vi "jsontest3.vi"() -> ()   [LabVIEW 2014]
panel:
  out "JSON string":string
  out "value 3":T1(array[cluster])
  in  "value 2":T1(array[cluster])=[{"DEPT"="Z", "LINE"="L2A", "STANO"="1", "WORKNO"="壓縮機", "PRODSN"="0DO1100587", "COMPNTID"="9SS064XGA21", "COMPNTLOT"="F0033", "COMPNTSN"="9SS064XGA21~20210520F0033949", "USEDQTY"=1, "OPDATE"="20211026082804", "OPUSER"="SYSTEM", "RECVDATE"="20211026082804", "MMODU"="KCI"}, {"DEPT"="Z", "LINE"="L2A", "STANO"="1", "WORKNO"="馬達", "PRODSN"="0DO1100587", "COMPNTID"="9SS064XGA21", "COMPNTLOT"="F0033", "COMPNTSN"="9SS064XGA21", "USEDQTY"=1, "OPDATE"="202110260828", "OPUSER"="SYSTEM", "RECVDATE"="202110260828", "MMODU"="KCI"}, {"DEPT"="Z", "LINE"="L2A", "STANO"="1", "WORKNO"="電源板", "PRODSN"="0DO1100587", "COMPNTID"="2", "COMPNTLOT"="3", "COMPNTSN"="4", "USEDQTY"=1, "OPDATE"="202110260828", "OPUSER"="SYSTEM", "RECVDATE"="202110260828", "MMODU"="KCI"}]
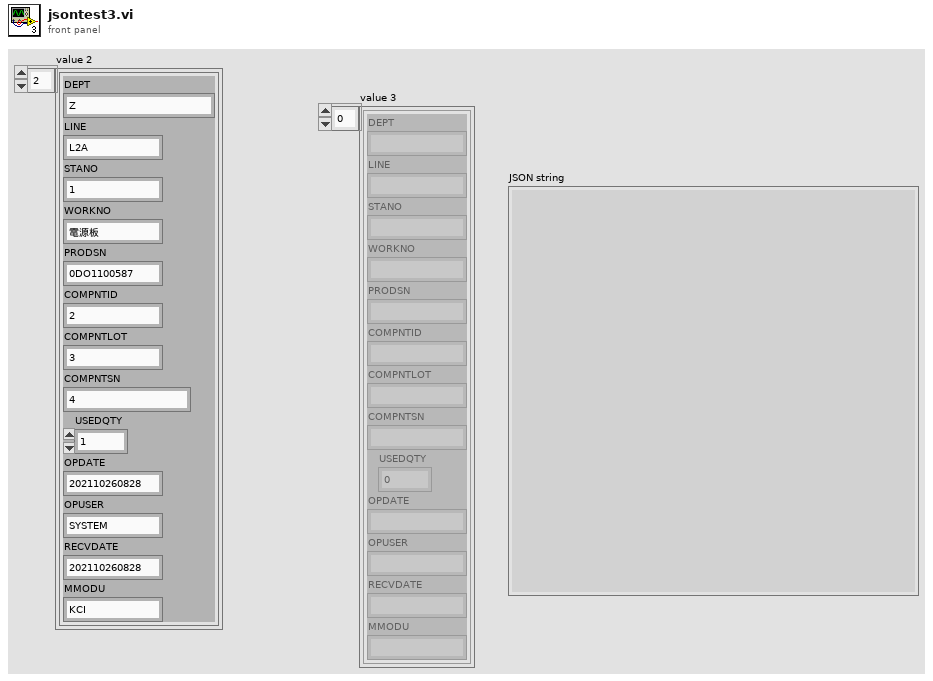
[diagram p1: front panel]
types:
  T1 = cluster{"DEPT":string, "LINE":string, "STANO":string, "WORKNO":string, "PRODSN":string, "COMPNTID":string, "COMPNTLOT":string, "COMPNTSN":string, "USEDQTY":i16, "OPDATE":string, "OPUSER":string, "RECVDATE":string, "MMODU":string}[]
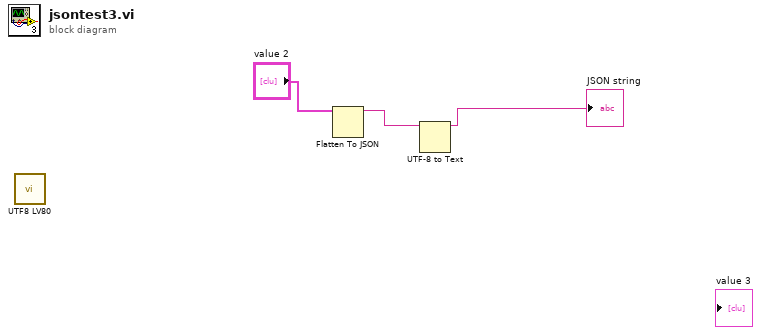
[diagram p0: block diagram]
diagram:
  n1 = call "UTF8 LV80.vi"() -> ()  [unwired: 1 in]
  n2 = Flatten To JSON(anything="value 2") -> (JSON string=w2:string)  [unwired: 2 in, 1 out]
  n3 = UTF-8 to Text(11:w2) -> (3:→"JSON string":string)  [unwired: 2 in, 1 out]
